vi "Create Route Path.vi"(8 "error in":errorcluster, 10 "Source":string, 11 "2525 in":refnum<class "2525.lvclass">) -> (0 "error out":errorcluster, 3 "2525 out":refnum<class "2525.lvclass">)   [LabVIEW 2019, in "2525.lvlib" / "2525.lvclass"]
uses:
  Library/2525.lvclass
  C:/Users/rdexter/Desktop/Built/SwitchMatrix.lvlibp/SwitchMatrix.lvclass
  Library/2525.lvclass/2525.ctl
  Accessors/Read Com Channels.vi
  Accessors/Read Modulo.vi
  builds/Instruments/SwitchMatrix.lvlibp/Accessors/Read Relay Name.vi
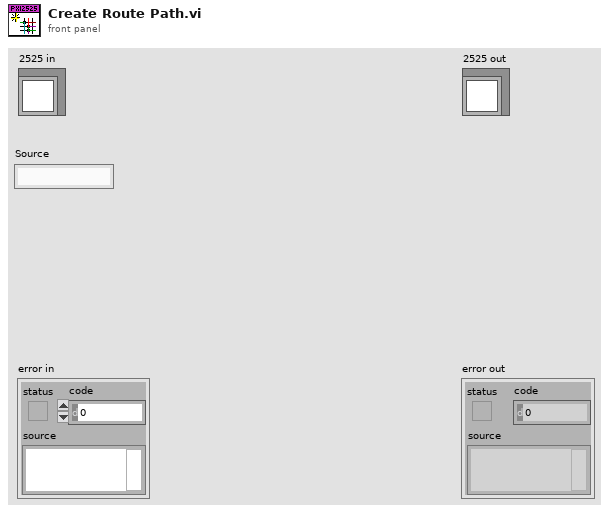
[diagram p1: front panel]
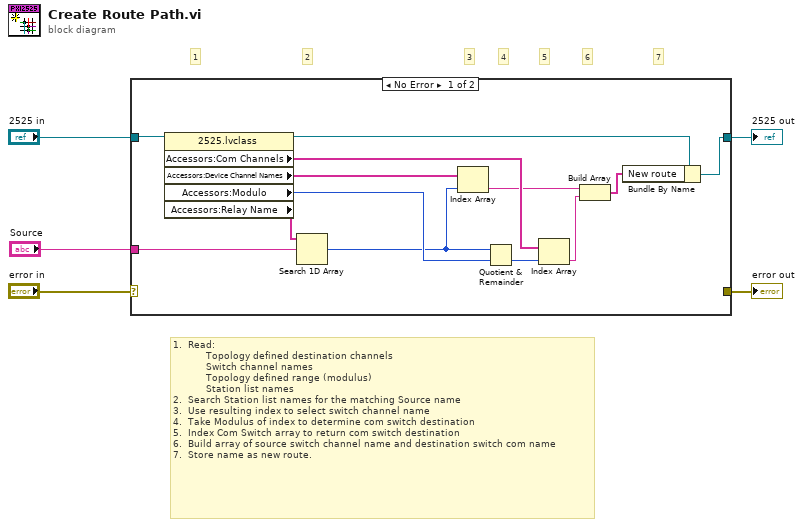
[diagram p0: block diagram]
diagram:
  # "7"
  # "1.  Read:\n           Topology defined destination channels\n           Switch channel names\n           Topology defined range (modulus)\n           Station list names\n2.  Search Station list names for the matching Source name\n3.  Use resulting index to select switch channel name\n4.  Take Modulus of index to determine com switch destination\n5.  Index Com Switch array to return com switch destination\n6.  Build array of source switch channel name and destination switch com name\n7.  Store name as new route."
  # "6"
  # "5"
  # "4"
  # "3"
  # "2"
  # "1"
  n1 = case shown="No Error" "error in" {
    selector: "error in" -> [_ w20]
    tunnel: [_ w20] -> w4
    tunnel: [w9 w19] -> w2
    tunnel: "2525 in" -> [w18 w19]
    tunnel: "Source" -> [w16 _]
    frame No Error {
      n2 = property class="2525.lvclass"(reference=w18) -> (reference out=w10:refnum<class "2525.lvclass">, "Accessors:Com Channels"=w11:string[], "Accessors:Device Channel Names"=w12:string[], "Accessors:Modulo"=w15:i32, "Accessors:Relay Name"=w17:string[])  [unwired: 1 in, 1 out]
      n3 = Search 1D Array(1D array=w17, element=w16) -> (index of element=w13:i32)  [unwired: 1 in]
      n4 = Index Array(array=w12, index=w13) -> (element=w8:string)
      n5 = Quotient & Remainder(x=w13, y=w15) -> (floor(x/y)=w14:i32)  [unwired: 1 out]
      n6 = Index Array(array=w11, index=w14) -> (element=w7:string)
      n7 = Build Array(w8, w7) -> (w6:string[])
      n8 = Bundle By Name(cluster=w10, "New route"=w6) -> (w9:refnum<class "2525.lvclass">)
    }
    frame Error {
    }
  }
  "error out" <- w4
  "2525 out" <- w2
